vi "NI 影像處理Barcode辨識.vi"() -> ()   [LabVIEW 2019]
panel:
  out "Barcode Grading Report (Barcode Reader 1)":T1(array[cluster])
  out "Complete Data (Barcode Reader 1)":string[](array[string])
  out "Barcodes (Barcode Reader 1)":T2(array[cluster]) {"Confidence Level" format="%.2f"; "Barcode Type" items=["Reserved", "Codabar", "Code 39", "Code 93", "Code 128", "EAN 8", "EAN 13", "Interleaved 2 of 5", "MSI", "UPCA", "Pharmacode", "RSS Limited"]; "Bounding Box"."y" format="%.2f"; "Bounding Box"."x" format="%.2f"}
  in  "stop":bool
  out "Image":T3(plugin-control)
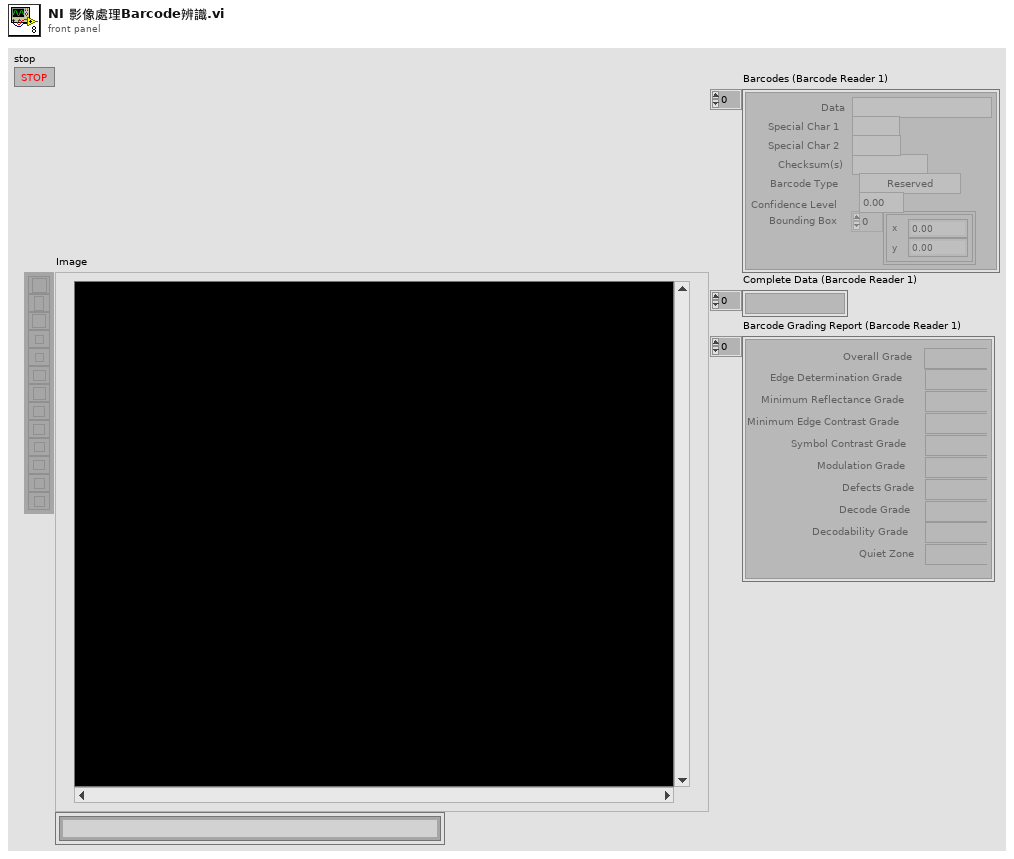
[diagram p1: front panel]
types:
  T1 = cluster{"Overall Grade":string, "Edge Determination Grade":string, "Minimum Reflectance Grade":string, "Minimum Edge Contrast Grade":string, "Symbol Contrast Grade":string, "Modulation Grade":string, "Defects Grade":string, "Decode Grade":string, "Decodability Grade":string, "Quiet Zone":string}[]
  T2 = cluster{"Data":string, "Special Char 1":string, "Special Char 2":string, "Checksum(s)":string, "Barcode Type":u32, "Confidence Level":sgl, "Bounding Box":cluster{"x":sgl, "y":sgl}[]}[]
  T3 = typedef "IMAQ Image.ctl" = refnum<image>
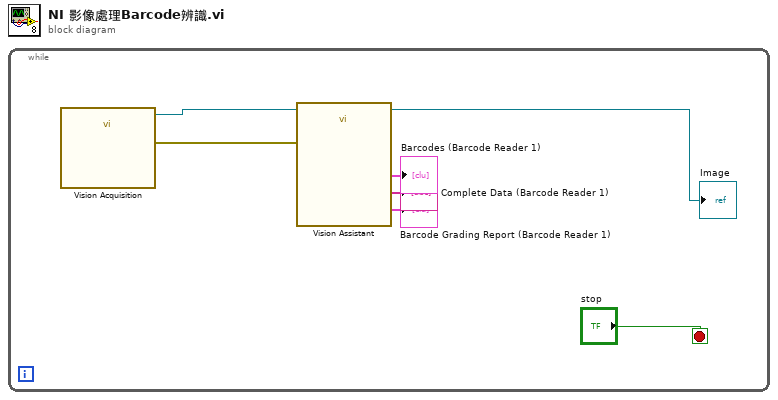
[diagram p0: block diagram]
diagram:
  n1 = while {
    stop <- "stop" stop-if-true
    n2 = call "Vision Acquisition"() -> ("Image Out"=w7:T3, "error out"=w6:errorcluster)  [unwired: 25 in, 1 out]
    n3 = call "Vision Assistant"("Image In"=w7, "error in"=w6) -> ("Image Out"=→"Image":T3, "Barcodes (Barcode Reader 1)"=→"Barcodes (Barcode Reader 1)":T2, "Complete Data (Barcode Reader 1)"=→"Complete Data (Barcode Reader 1)":string[], "Barcode Grading Report (Barcode Reader 1)"=→"Barcode Grading Report (Barcode Reader 1)":T1)  [unwired: 21 in, 1 out]
  }
